vi "Zero pad array (SubVI).vi"(10 "length":i32, 11 "Array in":dbl[](array[numeric])) -> (3 "Array out":dbl[](array[numeric]))   [LabVIEW 2011]
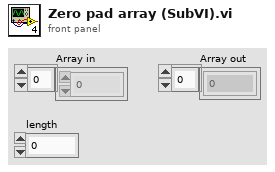
[diagram p1: front panel]
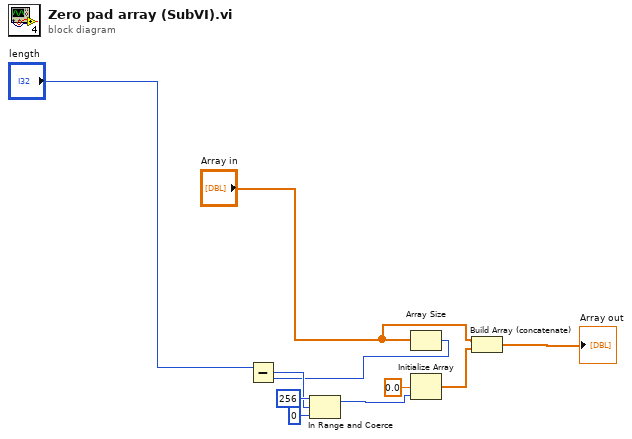
[diagram p0: block diagram]
diagram:
  n1 = Array Size(array="Array in") -> (size(s)=w2:i32)
  n2 = Subtract(x="length", y=w2) -> (x-y=w6:i32)
  n3 = In Range and Coerce(upper limit=256, x=w6, lower limit=0) -> (coerced(x)=w8:i32)  [unwired: 1 out]
  n4 = Initialize Array(0.0 ("element"), w8) -> (w5:dbl[])
  n5 = Build Array (concatenate)("Array in", w5) -> (→"Array out":dbl[])
